vi "capabilities.vi"(7 "LabVIEW Web Service Request":refnum<class "Web Request.lvclass">, 11 "context_id":string) -> (3 "capabilities":string[](array[string]))   [LabVIEW 2013]
uses:
  <vilib>/wsapi/Web Request.lvclass
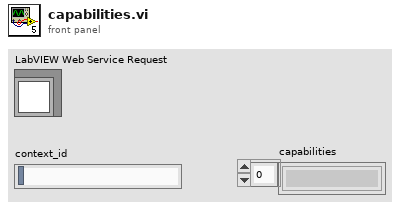
[diagram p1: front panel]
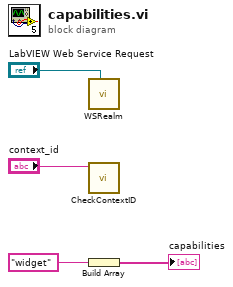
[diagram p0: block diagram]
diagram:
  n1 = call "WSRealm.vi"("LabVIEW Web Service Request"="LabVIEW Web Service Request") -> ()  [unwired: 11 in]
  n2 = call "CheckContextID.vi"("context_id"="context_id") -> ()  [unwired: 10 in, 1 out]
  n3 = Build Array("widget") -> (→"capabilities":string[])
